vi "Check Amplitude Offset Bounds.vi"(4 "Debug Message FIFO":refnum<k33>, 6 "MinV":dbl, 7 "Last Iter In Bounds?":bool, 8 "error in (no error)":errorcluster, 9 "MaxV":dbl, 10 "Offset":dbl, 11 "Amplitude":dbl) -> (0 "error out":errorcluster, 1 "Coerced Offset":dbl, 2 "Values In Bounds?":bool, 3 "Coerced Amplitude":dbl)   [LabVIEW 2023, in "Waveform Analog Output Engine.lvlib"]
uses:
  Waveform Analog Output Engine.lvlib
  Console Message Type.ctl
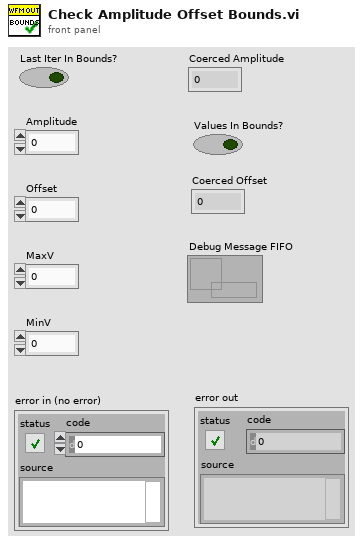
[diagram p1: front panel]
types:
  T1 = typedef "Waveform Analog Output Engine.lvlib/Console Message Type.ctl" = enum16{"Range Warning", "Error"}
  T2 = cluster{"Hw Max":dbl, "Hw Min":dbl, "Requested Amplitude":dbl, "Requested Offset":dbl, "Coerced Amplitude":dbl, "Coerced Offset":dbl}
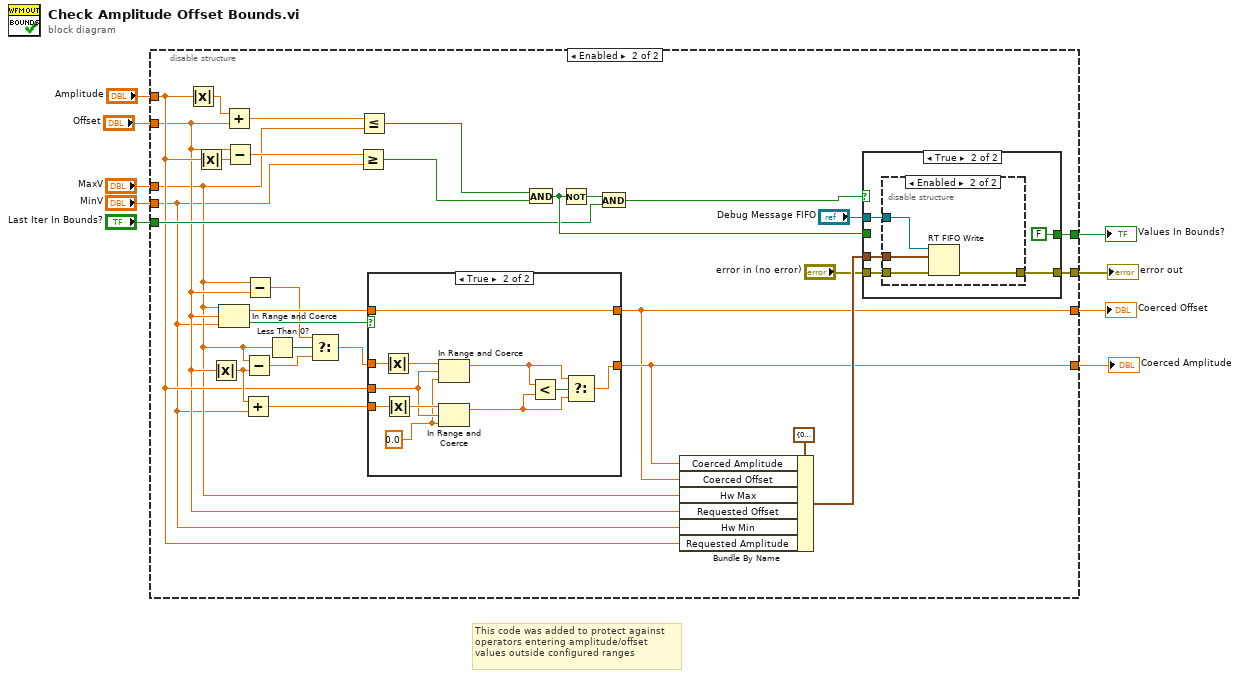
[diagram p0: block diagram]
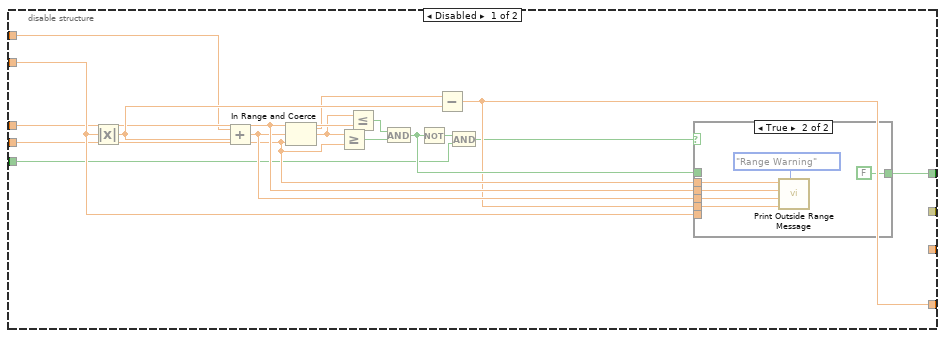
[diagram p2: hidden frame]
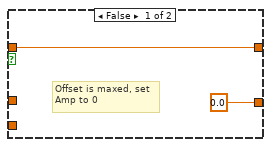
[diagram p4: hidden frame]
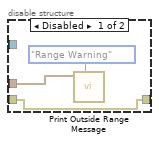
[diagram p6: hidden frame]
diagram:
  # "This code was added to protect against\noperators entering amplitude/offset\nvalues outside configured ranges"
  n1 = disable-structure shown="Enabled" {
    disable-tunnel: "Offset" -> [w24 w36]
    disable-tunnel: "MaxV" -> [w19 w35]
    disable-tunnel: "MinV" -> [w17 w34]
    disable-tunnel: [w16 w39] -> w6
    disable-tunnel: "Amplitude" -> [w14 w47]
    disable-tunnel: [w13 w61] -> w4
    disable-tunnel: "Last Iter In Bounds?" -> [w11 w60]
    disable-tunnel: [_ w38] -> w2
    disable-tunnel: [_ w40] -> w1
    frame Disabled {
      n2 = Absolute Value(x=w24) -> (abs(x)=w23:dbl)
      n3 = Add(x=w14, y=w23) -> (x+y=w18:dbl)
      n4 = In Range and Coerce(upper limit=w19, x=w18, lower limit=w17) -> (coerced(x)=w15:dbl)  [unwired: 1 out]
      n5 = Greater Or Equal?(x=w18, y=w17) -> (x >= y?=w21:bool)
      n6 = Less Or Equal?(x=w18, y=w19) -> (x <= y?=w20:bool)
      n7 = And(x=w20, y=w21) -> (x .and. y?=w22:bool)
      n8 = Not(x=w22) -> (.not. x?=w10:bool)
      n9 = Subtract(x=w15, y=w23) -> (x-y=w16:dbl)
      n10 = And(x=w10, y=w11) -> (x .and. y?=w12:bool)
      n11 = case shown="True" w12 {
        tunnel: w17 -> [_ w32]
        tunnel: w19 -> [_ w31]
        tunnel: w18 -> [_ w30]
        tunnel: w16 -> [_ w29]
        tunnel: w22 -> [w25 _]
        tunnel: [w25 FALSE] -> w13
        tunnel: w24 -> [_ w26]
        frame False {
        }
        frame True {
          n12 = call "Print Outside Range Message.vi"(4:w26, 6:w29, "Message Type"=Console_Message_Type."Range Warning", 9:w30, 10:w31, "Message Values"=w32) -> ()  [unwired: 6 in]
        }
      }
    }
    frame Enabled {
      n13 = Absolute Value(x=w47) -> (abs(x)=w37:dbl)
      n14 = Absolute Value(x=w47) -> (abs(x)=w48:dbl)
      n15 = Absolute Value(x=w36) -> (abs(x)=w52:dbl)
      n16 = In Range and Coerce(upper limit=w35, x=w36, lower limit=w34) -> (coerced(x)=w53:dbl, In Range?=w54:bool)
      n17 = Add(x=w37, y=w36) -> (x+y=w58:dbl)
      n18 = Subtract(x=w36, y=w48) -> (x-y=w57:dbl)
      n19 = Add(x=w52, y=w34) -> (x+y=w51:dbl)
      n20 = Subtract(x=w35, y=w52) -> (x-y=w45:dbl)
      n21 = Subtract(x=w35, y=w36) -> (x-y=w44:dbl)
      n22 = Less Than 0?(x=w35) -> (x < 0?=w46:bool)
      n23 = Select(t=w44, s=w46, f=w45) -> (s? t:f=w43:dbl)
      n24 = Greater Or Equal?(x=w57, y=w34) -> (x >= y?=w55:bool)
      n25 = Less Or Equal?(x=w58, y=w35) -> (x <= y?=w56:bool)
      n26 = case shown="True" w54 {
        tunnel: w53 -> [w64 w75]
        tunnel: [w64 w75] -> w38
        tunnel: [0.0 ("Coerced Amplitude") w67] -> w39
        tunnel: w43 -> [_ w74]
        tunnel: w51 -> [_ w73]
        tunnel: w47 -> [_ w70]
        frame False {
          # "Offset is maxed, set\nAmp to 0"
        }
        frame True {
          w69 = 0.0
          n27 = Absolute Value(x=w74) -> (abs(x)=w72:dbl)
          n28 = Absolute Value(x=w73) -> (abs(x)=w71:dbl)
          n29 = In Range and Coerce(upper limit=w72, x=w70, lower limit=w69) -> (coerced(x)=w65:dbl)  [unwired: 1 out]
          n30 = In Range and Coerce(upper limit=w71, x=w70, lower limit=w69) -> (coerced(x)=w66:dbl)  [unwired: 1 out]
          n31 = Less?(x=w65, y=w66) -> (x < y?=w68:bool)
          n32 = Select(t=w65, s=w68, f=w66) -> (s? t:f=w67:dbl)
        }
      }
      n33 = And(x=w56, y=w55) -> (x .and. y?=w62:bool)
      n34 = Not(x=w62) -> (.not. x?=w59:bool)
      n35 = And(x=w59, y=w60) -> (x .and. y?=w33:bool)
      n36 = Bundle By Name(cluster=T2 {"Hw Max"=0.0, "Hw Min"=0.0, "Requested Amplitude"=0.0, "Requested Offset"=0.0, "Coerced Amplitude"=0.0, "Coerced Offset"=0.0} ("Message Values"), "Coerced Amplitude"=w39, "Coerced Offset"=w38, "Hw Max"=w35, "Requested Offset"=w36, "Hw Min"=w34, "Requested Amplitude"=w47) -> (w49:T2)
      n37 = case shown="True" w33 {
        tunnel: w62 -> [w77 _]
        tunnel: [w77 FALSE] -> w61
        tunnel: w49 -> [_ w81]
        tunnel: "Debug Message FIFO" -> [_ w80]
        tunnel: "error in (no error)" -> [w76 w79]
        tunnel: [w76 w78] -> w40
        frame False {
        }
        frame True {
          n38 = disable-structure shown="Enabled" {
            disable-tunnel: w81 -> [w84 w88]
            disable-tunnel: w80 -> [_ w89]
            disable-tunnel: w79 -> [w83 w87]
            disable-tunnel: [w83 w86] -> w78
            frame Disabled {
              n39 = call "Print Outside Range Message.vi"("Message Type"=Console_Message_Type."Range Warning", "Message Values"=w84) -> ()  [unwired: 10 in]
            }
            frame Enabled {
              n40 = RT FIFO Write(0:w89, 1:w88, 3:w87) -> (11:w86:errorcluster)  [unwired: 2 in, 3 out]
            }
          }
        }
      }
    }
  }
  "Coerced Amplitude" <- w6
  "Values In Bounds?" <- w4
  "Coerced Offset" <- w2
  "error out" <- w1
